vi "Get Sun Declination Angle.vi"(10 "Sun App Long (deg)":dbl, 11 "Oblique Correction (deg)":dbl) -> (3 "Numeric":dbl)   [LabVIEW 2014, in "Solar Calculations.lvlib"]
uses:
  Solar Calculations.lvlib
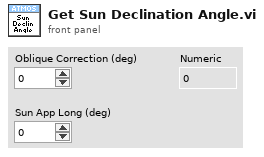
[diagram p1: front panel]
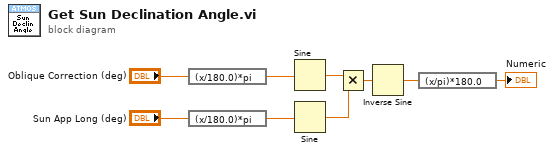
[diagram p0: block diagram]
diagram:
  n1 = expression code="(x/180.0)*pi" ("degrees to radians")("Oblique Correction (deg)") -> (w3:dbl)
  n2 = expression code="(x/180.0)*pi" ("degrees to radians")("Sun App Long (deg)") -> (w2:dbl)
  n3 = Sine(x=w3) -> (sin(x)=w6:dbl)
  n4 = Sine(x=w2) -> (sin(x)=w5:dbl)
  n5 = Multiply(x=w6, y=w5) -> (x*y=w7:dbl)
  n6 = Inverse Sine(1:w7) -> (0:w8:dbl)
  n7 = expression code="(x/pi)*180.0" ("radians to degrees")(w8) -> (→"Numeric":dbl)
